vi "CreatePublicEvents.vi"(8 "error in (no error)":errorcluster, 11 "XYStage":refnum<class "XYStage.lvclass">) -> (0 "error out":errorcluster, 3 "XYStage out":refnum<class "XYStage.lvclass">)   [LabVIEW 2017, in "XYStage.lvclass"]
doc: "---------------------------------------------------------------\nJKI State Machine Objects™\nhttp://jki.net/state-machine-objects/\nCopyright (C) 2005-2015, JKI <info@jki.net>\nALL RIGHTS RESERVEDJKI State Machine Objects (SMO) 1.0.0.5\nJKI - JKI\nCopyright (c) 2016, JKI"
uses:
  XYStage.lvclass
  XYStage.lvclass/XYStage.ctl
  Typedefs/PublicEvents--XYStage.StatusUpdated.ctl
  Typedefs/XYStage.Axis--Enum.ctl
  Typedefs/XYStage.DeviceStatus--Enum.ctl
  Device/Device.lvclass
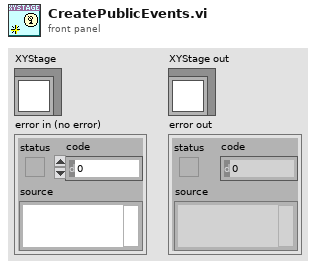
[diagram p1: front panel]
types:
  T1 = typedef "XYStage.lvclass/PrivateData--Ref.ctl" = refnum<data-value>
  T2 = typedef "XYStage.lvclass/PublicEvents--XYStage.StatusUpdated.ctl" = cluster{"Axis":T3, "Position":i32, "IsEnabled":bool, "IsError":bool, "IsMoving":bool, "Status":T4}
  T3 = typedef "XYStage.lvclass/XYStage.Axis--Enum.ctl" = u16
  T4 = typedef "XYStage.lvclass/XYStage.DeviceStatus--Enum.ctl" = u32
  T5 = typedef "XYStage.lvclass/PrivateData--Cluster.ctl" = cluster{"Configuration":T6, "Public Events":T7, "Protected Events":T8, "Data":string}
  T6 = typedef "XYStage.lvclass/Configuration--Cluster.ctl" = cluster{"Serial Number":string, "X Axis":string, "Y Axis":string, "Real-World Units":string, "Counts per Unit":dbl}
  T7 = typedef "XYStage.lvclass/PublicEvents--Cluster.ctl" = cluster{"StatusUpdated":refnum<user-event>}
  T8 = typedef "XYStage.lvclass/ProtectedEvents--Cluster.ctl" = cluster{"API_Template":refnum<user-event>}
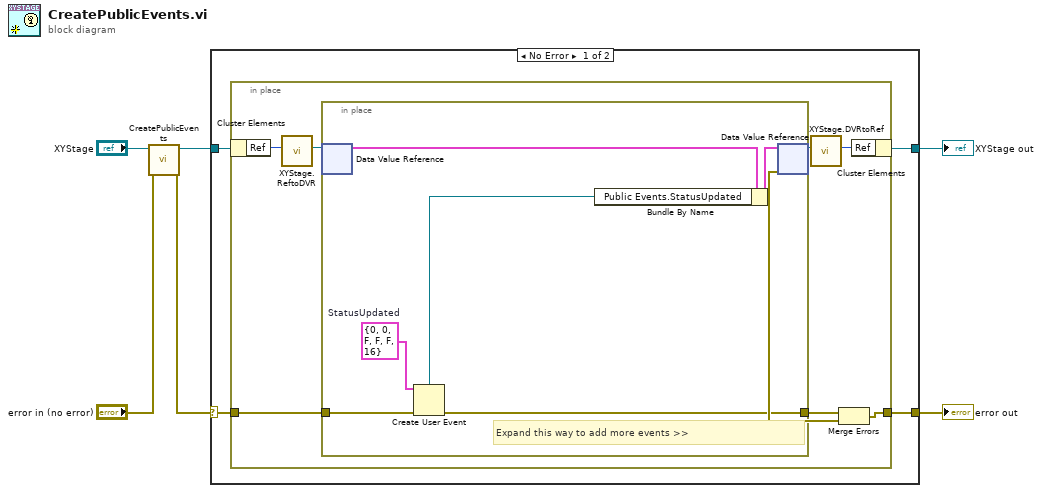
[diagram p0: block diagram]
diagram:
  n1 = call-parent "CreatePublicEvents.vi"("error in (no error)"="error in (no error)", "Device"="XYStage") -> ("error out"=w1:errorcluster, "Device out"=w3:refnum<class "XYStage.lvclass">)  [unwired: 8 in]
  n2 = case shown="No Error" w1 {
    selector: w1 -> [w8 w26]
    tunnel: [w7 w26] -> w5
    tunnel: [w9 w25] -> w6
    tunnel: w3 -> [w10 w25]
    frame No Error {
      n3 = in-place {
        in-place-border: w8 -> [w18]
        in-place-border: [w15] -> w7
        n4 = in-place-cluster #1(w10) -> ("Ref"=w14:u32)
        n5 = call "XYStage.ReftoDVR.vi"("Ref"=w14) -> ("Ref"=w13:T1)  [unwired: 10 in]
        n6 = in-place {
          in-place-border: w18 -> [w22]
          in-place-border: [w21] -> w17
          w20 = T2 {"Axis"=0, "Position"=0, "IsEnabled"=FALSE, "IsError"=FALSE, "IsMoving"=FALSE, "Status"=16}  # StatusUpdated
          # "Expand this way to add more events >>"
          n7 = in-place-dvr #2(w13) -> (w23:T5)  [unwired: 1 out]
          n8 = Create User Event(user event datatype=w20, error in=w22) -> (user event=w19:refnum<user-event>, error out=w21:errorcluster)
          n9 = Bundle By Name(cluster=w23, "Public Events.StatusUpdated"=w19) -> (w24:T5)
          n10 = in-place-dvr #2(w24) -> (w12:T1, w16:errorcluster)
        }
        n11 = call "XYStage.DVRtoRef.vi"("Ref"=w12) -> ("Ref"=w11:u32)  [unwired: 10 in]
        n12 = Merge Errors(w17, w16) -> (w15:errorcluster)
        n13 = in-place-cluster #1("Ref"=w11) -> (w9:refnum<class "XYStage.lvclass">)
      }
    }
    frame Error {
    }
  }
  "error out" <- w5
  "XYStage out" <- w6
